vi "dsPIC Test.vi"() -> ()   [LabVIEW 2018]
panel:
  in  "HV Set Point 2":u8
  in  "Temp Set Point":u8
  in  "PIC Number":u8
  # "CORONA dsPIC33"
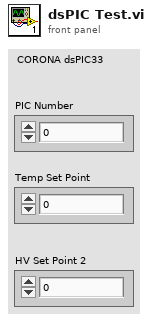
[diagram p1: front panel]
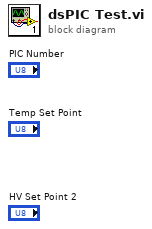
[diagram p0: block diagram]
diagram:
